vi "SalvarInformacoesRelatorio.vi"() -> (0 "error out":errorcluster, 3 "NomeDocumento":string)   [LabVIEW 2019]
uses:
  21e89efe-00a0-40b3-80f4-28f26c716dbc.vi
  VariaveisMedicao.vi
  Relatorio/Relatorio_Variaveis.vi
  TelaConfig/Configuracao.Variaveis.vi
  Relatorio/SalvarDadosTemporario.vi
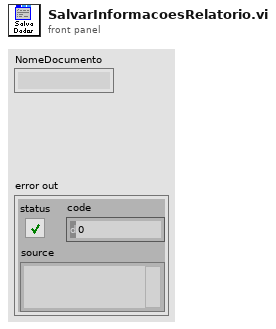
[diagram p1: front panel]
types:
  T1 = cluster{"Graph":cluster{"Descricao":string, "Graph":cluster{"X":dbl, "Y":dbl}[]}[], "Data":timestamp, "ModeloMotor":string, "ModeloInversor":string, "ModeloAeroGerador":string, "PotenciaAero":string}
  T2 = cluster{"Descricao":string, "Graph":cluster{"X":dbl, "Y":dbl}[]}
  T3 = cluster{"Descricao":string, "Graph":cluster{"X":dbl, "Y":dbl}[]}[]
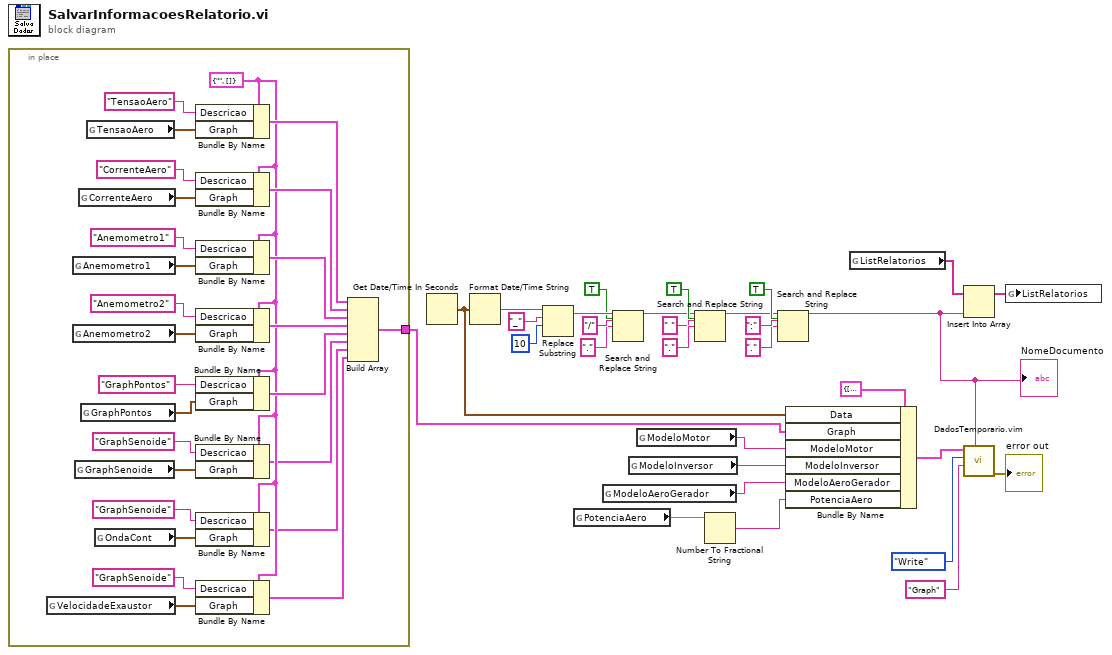
[diagram p0: block diagram]
diagram:
  n1 = in-place {
    in-place-border: [w31] -> w26
    w35 = T2 {"Descricao"="", "Graph"=[]} ("Cluster")
    n2 = global read "VariaveisMedicao.vi" "VelocidadeExaustor"() -> (w36:cluster{"X":dbl, "Y":dbl}[])
    n3 = global read "VariaveisMedicao.vi" "Anemometro1"() -> (w43:cluster{"X":dbl, "Y":dbl}[])
    n4 = global read "VariaveisMedicao.vi" "Anemometro2"() -> (w42:cluster{"X":dbl, "Y":dbl}[])
    n5 = global read "VariaveisMedicao.vi" "GraphSenoide"() -> (w40:cluster{"X":dbl, "Y":dbl}[])
    n6 = global read "VariaveisMedicao.vi" "CorrenteAero"() -> (w49:cluster{"X":dbl, "Y":dbl}[])
    n7 = global read "VariaveisMedicao.vi" "GraphPontos"() -> (w41:cluster{"X":dbl, "Y":dbl}[])
    n8 = global read "VariaveisMedicao.vi" "TensaoAero"() -> (w55:cluster{"X":dbl, "Y":dbl}[])
    n9 = global read "VariaveisMedicao.vi" "OndaCont"() -> (w37:cluster{"X":dbl, "Y":dbl}[])
    n10 = Bundle By Name(cluster=w35, "Descricao"="TensaoAero", "Graph"=w55) -> (w48:T2)
    n11 = Bundle By Name(cluster=w35, "Descricao"="CorrenteAero", "Graph"=w49) -> (w47:T2)
    n12 = Bundle By Name(cluster=w35, "Descricao"="Anemometro1", "Graph"=w43) -> (w46:T2)
    n13 = Bundle By Name(cluster=w35, "Descricao"="Anemometro2", "Graph"=w42) -> (w45:T2)
    n14 = Bundle By Name(cluster=w35, "Descricao"="GraphPontos", "Graph"=w41) -> (w44:T2)
    n15 = Bundle By Name(cluster=w35, "Descricao"="GraphSenoide", "Graph"=w40) -> (w34:T2)
    n16 = Bundle By Name(cluster=w35, "Descricao"="GraphSenoide", "Graph"=w37) -> (w33:T2)
    n17 = Bundle By Name(cluster=w35, "Descricao"="GraphSenoide", "Graph"=w36) -> (w32:T2)
    n18 = Build Array(w48, w47, w46, w45, w44, w34, w33, w32) -> (w31:T3)
  }
  n19 = Get Date/Time In Seconds() -> (seconds since 1Jan1904=w27:timestamp)
  n20 = Format Date/Time String(seconds (now)=w27) -> (date/time string=w22:string)  [unwired: 2 in]
  n21 = Replace Substring(3:10 ("offset (0)"), 4:"_" ("substring (\"\")"), 5:w22) -> (1:w19:string)  [unwired: 1 in, 1 out]
  n22 = global read "Configuracao.Variaveis.vi" "PotenciaAero"() -> (w2:dbl)
  n23 = global read "Configuracao.Variaveis.vi" "ModeloAeroGerador"() -> (w3:string)
  n24 = Search and Replace String(replace all?=TRUE ("replace all? (F)"), input string=w19, search string="/", replace string="." ("replace string (\"\")")) -> (result string=w9:string)  [unwired: 4 in, 3 out]
  n25 = global read "Configuracao.Variaveis.vi" "ModeloInversor"() -> (w4:string)
  n26 = global read "Configuracao.Variaveis.vi" "ModeloMotor"() -> (w5:string)
  n27 = Search and Replace String(replace all?=TRUE ("replace all? (F)"), input string=w9, search string=" ", replace string="." ("replace string (\"\")")) -> (result string=w8:string)  [unwired: 4 in, 3 out]
  n28 = Number To Fractional String(number=w2) -> (F-format string=w1:string)  [unwired: 3 in]
  n29 = Search and Replace String(replace all?=TRUE ("replace all? (F)"), input string=w8, search string=":", replace string="." ("replace string (\"\")")) -> (result string=w7:string)  [unwired: 4 in, 3 out]
  "NomeDocumento" <- w7
  n30 = Bundle By Name(cluster=T1 {"Graph"=[], "Data"=timestamp(3705620400 s since 1904-01-01), "ModeloMotor"="", "ModeloInversor"="", "ModeloAeroGerador"="", "PotenciaAero"=""} ("Cluster"), "Data"=w27, "Graph"=w26, "ModeloMotor"=w5, "ModeloInversor"=w4, "ModeloAeroGerador"=w3, "PotenciaAero"=w1) -> (w28:T1)
  n31 = global read "Relatorio_Variaveis.vi" "ListRelatorios"() -> (w24:string[])
  n32 = Insert Into Array(array=w24, new element=w7) -> (w23:string[])  [unwired: 1 in]
  n33 = call "DadosTemporario.vim"("FileName"=w7, "Directory"="Graph", "Read/Write(Read)"=enum16{"Read", "Write"}."Write", "DataInp"=w28) -> ("ErrorOut"=→"error out":errorcluster)  [unwired: 6 in, 1 out]
  n34 = global write "Relatorio_Variaveis.vi" "ListRelatorios"(w23) -> ()
